vi "GetPosition.vi"(8 "error in (no error)":errorcluster, 11 "3D Scene in":refnum<class "3D Scene.lvclass">) -> (0 "error out":errorcluster, 2 "Position":T1, 3 "3D Scene out":refnum<class "3D Scene.lvclass">)   [LabVIEW 2015, in "3D Scene.lvclass"]
uses:
  3D Scene.lvclass
  3D Point.ctl
  3D Scene.lvclass/3D Scene.ctl
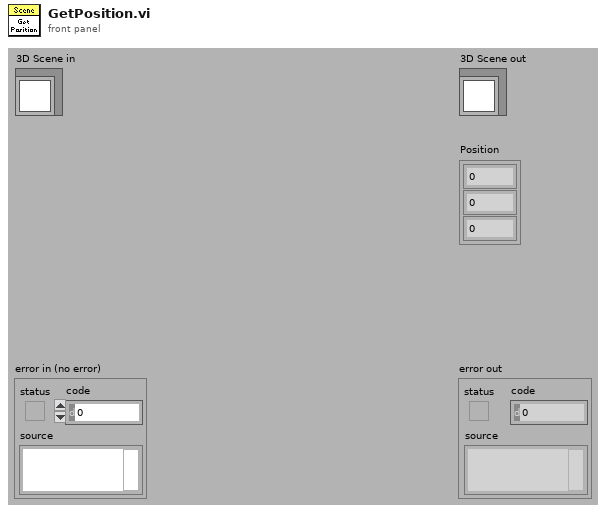
[diagram p1: front panel]
types:
  T1 = typedef "3D Point.ctl" = cluster{"X":sgl, "Y":sgl, "Z":sgl}
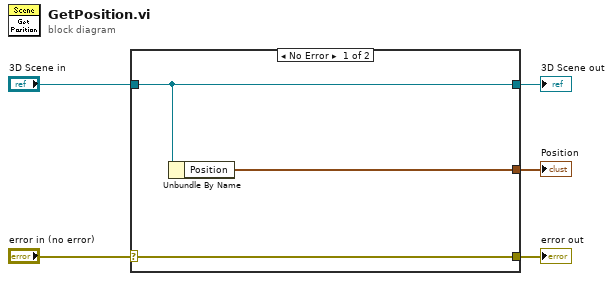
[diagram p0: block diagram]
diagram:
  n1 = case shown="No Error" "error in (no error)" {
    selector: "error in (no error)" -> [w8 w9]
    tunnel: [w8 w9] -> w4
    tunnel: [w7 w10] -> w2
    tunnel: "3D Scene in" -> [w7 w10]
    tunnel: [w6 _] -> w1
    frame No Error {
      n2 = Unbundle By Name(w7) -> ("Position"=w6:T1)
    }
    frame Error {
    }
  }
  "error out" <- w4
  "3D Scene out" <- w2
  "Position" <- w1
